vi "StopAcquisition.vi"(8 "error in (no error)":errorcluster, 11 "Microscope in":refnum<class "Microscope.lvclass">) -> (0 "error out":errorcluster, 3 "Microscope out":refnum<class "Microscope.lvclass">)   [LabVIEW 2020, in "Microscope.lvlib" / "Microscope.lvclass"]
uses:
  Microscope.lvclass
  Microscope.lvclass/Microscope.ctl
  <vilib>/ActorFramework/Message Enqueuer/Message Enqueuer.lvclass/Message Enqueuer.ctl
  <vilib>/ActorFramework/Message Enqueuer/Enqueue.vi
  Component/Device/Device Messages/StopAcquisition Msg/StopAcquisition Msg.lvclass
  C:/Program Files/National Instruments/LabVIEW 2020/vi.lib/ActorFramework/Message/Message.lvclass
  <vilib>/ActorFramework/Message Priority Queue/Priority Enqueue.vi
  Component/Device/Device/Device.lvclass
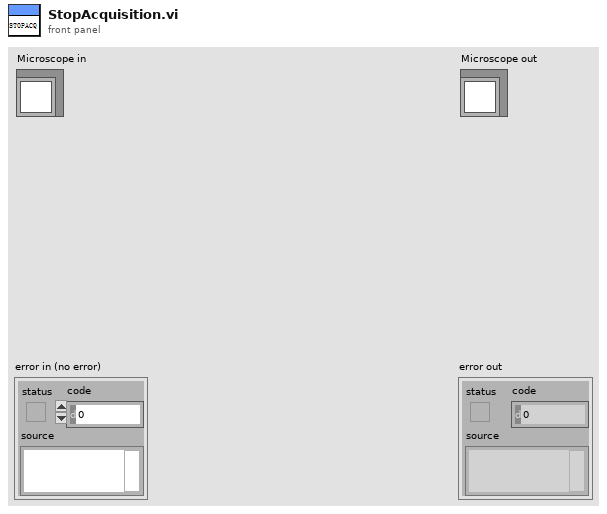
[diagram p1: front panel]
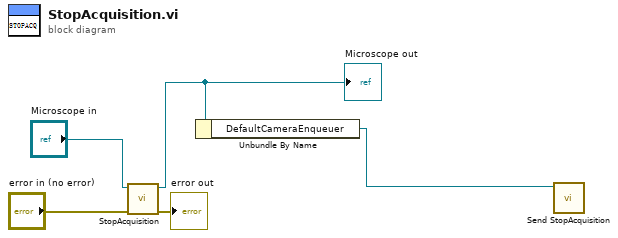
[diagram p0: block diagram]
diagram:
  n1 = call-parent "StopAcquisition.vi"("error in (no error)"="error in (no error)", "Device in"="Microscope in") -> ("error out"=→"error out":errorcluster, "Device out"=w2:refnum<class "Microscope.lvclass">)  [unwired: 8 in]
  "Microscope out" <- w2
  n2 = Unbundle By Name(w2) -> ("DefaultCameraEnqueuer"=w1:refnum<class "Message Enqueuer.lvclass">)
  n3 = call "Send StopAcquisition.vi"("Message Enqueuer"=w1) -> ()  [unwired: 9 in, 2 out]
